vi "edit io channel.vi"(6 "refresh UI":T2, 8 "error in":errorcluster, 9 "line":T1, 10 "engine configuration in":refnum<class "engine configuration.lvclass">, 11 "tag bus configurable plugin module configuration in":refnum<class "tag bus configurable plugin module configuration.lvclass">) -> (0 "error out":errorcluster, 1 "change?":bool, 2 "engine configuration":refnum<class "engine configuration.lvclass">, 3 "tag bus configurable plugin module configuration out":refnum<class "tag bus configurable plugin module configuration.lvclass">)   [LabVIEW 2013, in "tag bus configurable plugin editor node.lvclass"]
uses:
  tag bus configurable plugin editor node.lvclass
  <vilib>/NI/Configuration Framework/Node/RefreshUIEvent.ctl
  <vilib>/NI/Module Execution Interface/Engine Configuration/engine configuration.lvclass
  module/configuration/tag bus configurable plugin module configuration.lvclass
  table line.ctl
  <vilib>/NI/Tag Bus Module Framework/channel/TBM channel.lvclass
  <vilib>/NI/Configuration Framework/serializable configuration/NISE_CEF_serializable configuration.lvclass/NISE_CEF_serializable configuration.ctl
  <vilib>/NI/Configuration Framework/serializable configuration/NISE_CEF_serializable configuration.lvclass
  <vilib>/NI/Tag Bus/tag/tag descriptor.lvclass/tag descriptor.ctl
  <vilib>/NI/Tag Bus/tag/tag descriptor.lvclass
  <vilib>/NI/Configuration Framework/Node/NISE_CEF_Node.lvclass
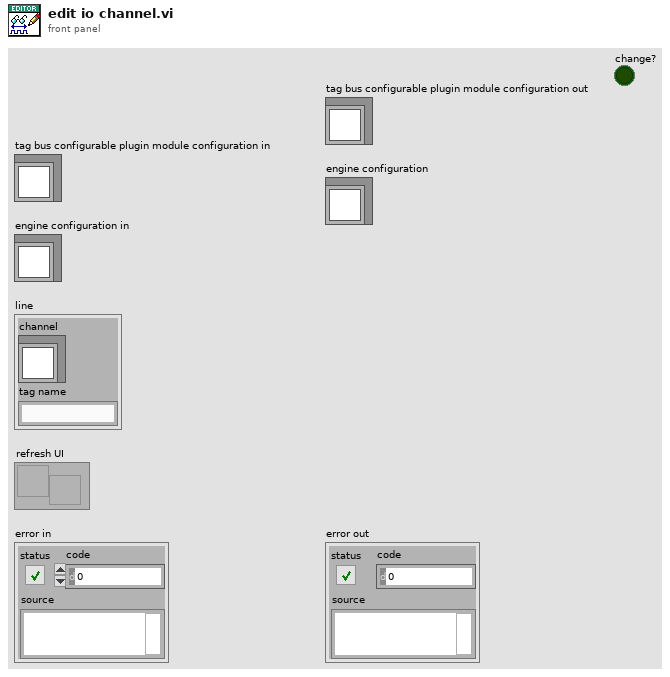
[diagram p1: front panel]
types:
  T1 = typedef "tag bus configurable plugin editor node.lvclass/table line.ctl" = cluster{"channel":refnum<class "TBM channel.lvclass">, "tag name":string}
  T2 = typedef "NISE_CEF_Node.lvclass/RefreshUIEvent.ctl" = refnum<user-event>
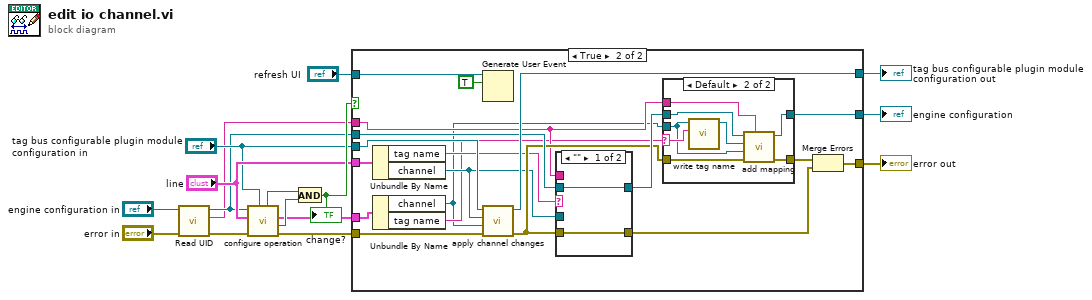
[diagram p0: block diagram]
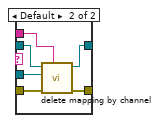
[diagram p4: hidden frame]
diagram:
  n1 = call <vilib>:"Read UID.vi"("error in"="error in", "configuration in"="engine configuration in") -> ("error out"=w4:errorcluster, "instance id"=w1:string, "configuration out"=w2:refnum<class "engine configuration.lvclass">)  [unwired: 7 in]
  n2 = call "configure operation.vi"("tag bus configurable plugin module configuration"="tag bus configurable plugin module configuration in", "error in"=w4, "line item in"="line", "engine configuration"=w2) -> ("error out"=w8:errorcluster, "success"=w12:bool, "line item out"=w9:T1, "changed"=w11:bool)  [unwired: 4 in]
  n3 = And(x=w11, y=w12) -> (x .and. y?=w13:bool)
  "change?" <- w13
  n4 = case shown="True" w13 {
    tunnel: [w18 w27] -> w6
    tunnel: [w19 w30] -> w15
    tunnel: w2 -> [w19 w32]
    tunnel: w8 -> [w18 w35]
    tunnel: w9 -> [_ w37]
    tunnel: "line" -> [_ w36]
    tunnel: "tag bus configurable plugin module configuration in" -> [w17 w38]
    tunnel: [w17 w33] -> w14
    tunnel: w1 -> [_ w23]
    tunnel: "refresh UI" -> [_ w34]
    frame False {
    }
    frame True {
      n5 = Unbundle By Name(w36) -> ("tag name"=w25:string, "channel"=w24:refnum<class "TBM channel.lvclass">)
      n6 = Unbundle By Name(w37) -> ("channel"=w21:refnum<class "TBM channel.lvclass">, "tag name"=w22:string)
      n7 = Generate User Event(user event=w34, event data cluster=TRUE ("event data")) -> ()  [unwired: 2 in, 2 out]
      n8 = call "apply channel changes.vi"("error in"=w35, "new channel"=w21, "old channel"=w24, "tag bus configurable plugin module configuration in"=w38) -> ("error out"=w26:errorcluster, "tag bus configurable plugin module configuration out"=w33:refnum<class "tag bus configurable plugin module configuration.lvclass">)  [unwired: 6 in]
      n9 = case shown="\"\"" w25 {
        tunnel: w23 -> [_ w56]
        tunnel: w32 -> [w50 w55]
        tunnel: [w50 w54] -> w31
        tunnel: [w49 w53] -> w29
        tunnel: w26 -> [w49 w52]
        tunnel: w24 -> [_ w51]
        frame "" {
        }
        frame Default {
          n10 = call <vilib>:"delete mapping by channel.vi"("owner ID"=w56, "error in"=w52, "channel"=w51, "engine configuration in"=w55) -> ("error out"=w53:errorcluster, "engine configuration out"=w54:refnum<class "engine configuration.lvclass">)  [unwired: 6 in]
        }
      }
      n11 = case shown="Default" w22 {
        selector: w22 -> [_ w42]
        tunnel: w31 -> [w40 w48]
        tunnel: [w40 w47] -> w30
        tunnel: [w39 w46] -> w28
        tunnel: w26 -> [w39 w45]
        tunnel: w23 -> [_ w44]
        tunnel: w21 -> [_ w41]
        frame "" {
        }
        frame Default {
          n12 = call <vilib>:"write tag name.vi"("name"=w42, "system tag in"=w41) -> ("system tag out"=w43:refnum<class "TBM channel.lvclass">)  [unwired: 8 in, 1 out]
          n13 = call <vilib>:"add mapping.vi"("owner ID"=w44, "error in"=w45, "channel"=w41, "tag descriptor"=w43, "engine configuration"=w48) -> ("error out"=w46:errorcluster, "engine configuration out"=w47:refnum<class "engine configuration.lvclass">)  [unwired: 5 in]
        }
      }
      n14 = Merge Errors(w28, w29) -> (w27:errorcluster)
    }
  }
  "engine configuration" <- w15
  "tag bus configurable plugin module configuration out" <- w14
  "error out" <- w6
